vi "GV-ZoomHorizontalDrag.vi"(7 "Gviewer in":refnum<class "Gviewer.lvclass">, 8 "error in (no error)":errorcluster, 10 "Coords":T1, 11 "pict in":picture) -> (0 "error out":errorcluster, 3 "pict out":picture)   [LabVIEW 2020, in "Gviewer.lvclass"]
doc: "Andre Koelewijn, 8 May 2021\n\nDraw the zoom window for Horizontal Area"
uses:
  Gviewer.lvclass
  <vilib>/Utility/miscctls.llb/LVPoint32TypeDef.ctl
  Gviewer.lvclass/Gviewer.ctl
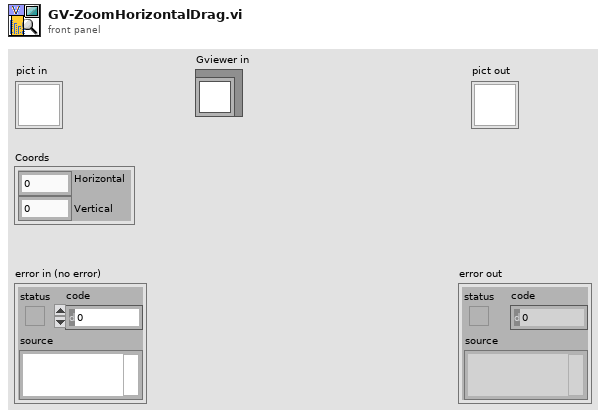
[diagram p1: front panel]
types:
  T1 = typedef "LVPoint32TypeDef.ctl" = cluster{"Horizontal":i32, "Vertical":i32}
  T2 = cluster{"Width":i16, "Style":enum32{"Solid", "Dash", "Dot", "DashDot", "DashDotDot"}}
  T3 = cluster{"left":i16, "top":i16, "right":i16, "bottom":i16}
  T4 = cluster{"horizontal":enum16{"left", "center", "right"}, "vertical":enum16{"top", "center", "bottom"}}
  T5 = typedef "LVRectTypeDef.ctl" = cluster{"Left":i16, "Top":i16, "Right":i16, "Bottom":i16}
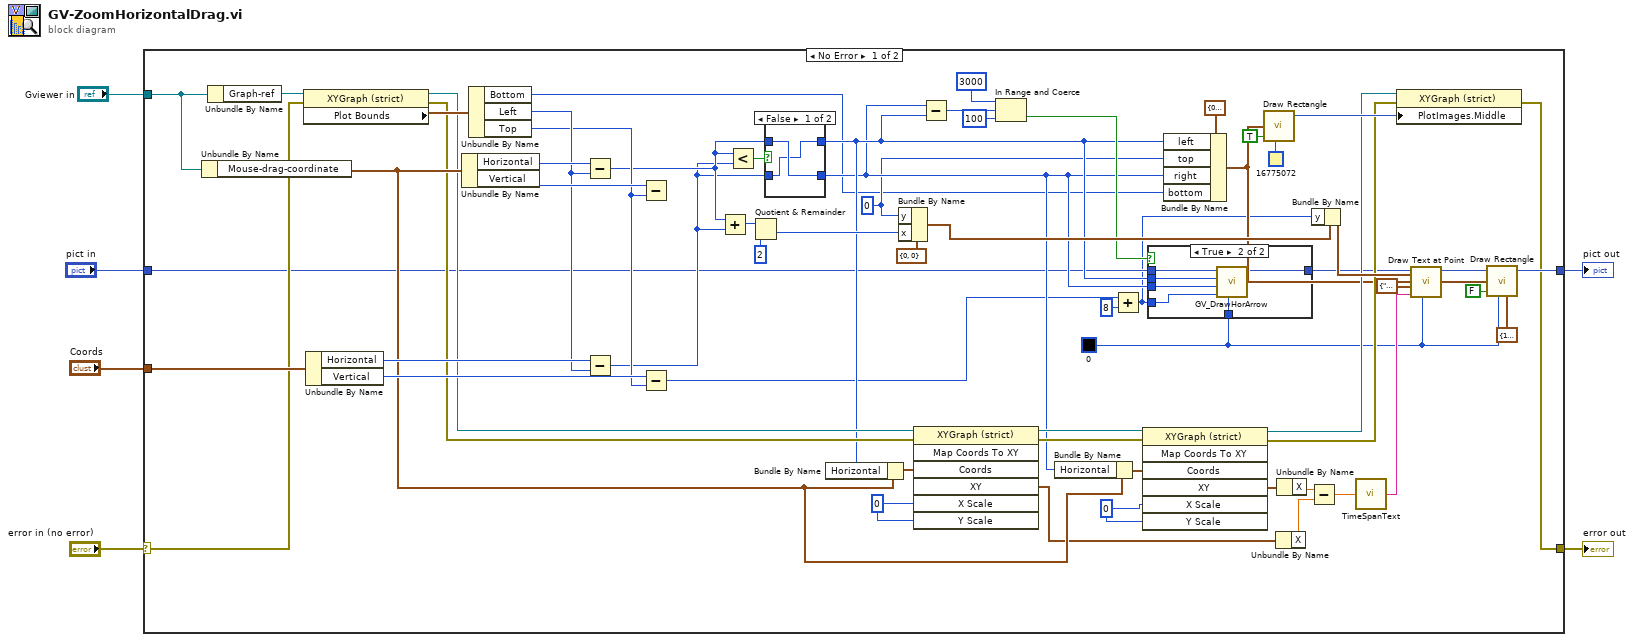
[diagram p0: block diagram]
diagram:
  n1 = case shown="No Error" "error in (no error)" {
    selector: "error in (no error)" -> [w40 w81]
    tunnel: [w28 w81] -> w5
    tunnel: "pict in" -> [w9 w80]
    tunnel: [w51 w80] -> w3
    tunnel: "Coords" -> [w67 _]
    tunnel: "Gviewer in" -> [w49 _]
    frame No Error {
      w10 = u32 0 ("Color")
      w12 = i16 0 ("top")
      w37 = 0 ("X Scale")
      w39 = 0 ("X Scale")
      n2 = Unbundle By Name(w49) -> ("Mouse-drag-coordinate"=w35:T1)
      n3 = Unbundle By Name(w49) -> ("Graph-ref"=w62:refnum<vi>)
      n4 = property class="XYGraph (strict)"(reference=w62, error in=w40) -> (reference out=w32:refnum<vi>, error out=w30:errorcluster, "Plot Bounds"=w61:T5)
      n5 = Unbundle By Name(w67) -> ("Horizontal"=w58:i32, "Vertical"=w56:i32)
      n6 = Unbundle By Name(w35) -> ("Horizontal"=w60:i32, "Vertical"=w59:i32)
      n7 = Unbundle By Name(w61) -> ("Bottom"=w11:i16, "Left"=w57:i16, "Top"=w55:i16)
      n8 = Subtract(x=w60, y=w57) -> (x-y=w48:i32)
      n9 = Subtract(x=w58, y=w57) -> (x-y=w47:i32)
      n10 = Subtract(x=w59, y=w55) -> ()  [unwired: 1 out]
      n11 = Subtract(x=w56, y=w55) -> (x-y=w8:i32)
      n12 = Add(x=w48, y=w47) -> (x+y=w46:i32)
      n13 = Less?(x=w48, y=w47) -> (x < y?=w54:bool)
      n14 = Quotient & Remainder(x=w46, y=2) -> (floor(x/y)=w43:i32)  [unwired: 1 out]
      n15 = case shown="False" w54 {
        tunnel: w48 -> [w77 w79]
        tunnel: [w76 w79] -> w15
        tunnel: [w77 w78] -> w14
        tunnel: w47 -> [w76 w78]
        frame False {
        }
        frame True {
        }
      }
      n16 = Bundle By Name(cluster=w35, "Horizontal"=w15) -> (w38:T1)
      n17 = Bundle By Name(cluster=cluster{"x":i16, "y":i16} {"x"=0, "y"=0} ("origin"), "y"=w12, "x"=w43) -> (w42:cluster{"x":i16, "y":i16})
      n18 = invoke class="XYGraph (strict)" method="Map Coords To XY"(reference=w32, error in=w30, "Coords"=w38, "X Scale"=w39, "Y Scale"=w39) -> (reference out=w36:refnum<vi>, error out=w33:errorcluster, "XY"=w25:cluster{"X":dbl, "Y":dbl})  [unwired: 2 in, 4 out]
      n19 = Subtract(x=w14, y=w15) -> (x-y=w20:i32)
      n20 = In Range and Coerce(upper limit=3000, x=w20, lower limit=100) -> (In Range?=w16:bool)  [unwired: 1 out]
      n21 = Bundle By Name(cluster=w35, "Horizontal"=w14) -> (w34:T1)
      n22 = Add(x=w8, y=8) -> (x+y=w7:i32)
      n23 = invoke class="XYGraph (strict)" method="Map Coords To XY"(reference=w36, error in=w33, "Coords"=w34, "X Scale"=w37, "Y Scale"=w37) -> (reference out=w31:refnum<vi>, error out=w29:errorcluster, "XY"=w27:cluster{"X":dbl, "Y":dbl})  [unwired: 2 in, 4 out]
      n24 = case shown="True" w16 {
        tunnel: w9 -> [w69 w75]
        tunnel: [w69 w74] -> w17
        tunnel: w15 -> [_ w73]
        tunnel: w14 -> [_ w72]
        tunnel: w7 -> [_ w71]
        tunnel: w10 -> [_ w70]
        frame False {
        }
        frame True {
          n25 = call "GV_DrawHorArrow.vi"("Color"=w70, "Vertical"=w71, "Right"=w72, "Left"=w73, "Pict-in"=w75) -> ("Pict-out"=w74:picture)  [unwired: 6 in]
        }
      }
      n26 = Bundle By Name(cluster=T3 {"left"=0, "top"=0, "right"=0, "bottom"=0} ("rect"), "left"=w15, "top"=w12, "right"=w14, "bottom"=w11) -> (w21:T3)
      n27 = call <vilib>:"Draw Rectangle.vi"("rect"=w21, "fill?(F)"=TRUE, "color(black)"=u32 16775072) -> ("new picture"=w66:picture)  [unwired: 6 in]
      n28 = Unbundle By Name(w25) -> ("X"=w24:dbl)
      n29 = Unbundle By Name(w27) -> ("X"=w26:dbl)
      n30 = Subtract(x=w26, y=w24) -> (x-y=w23:dbl)
      n31 = Bundle By Name(cluster=w42, "y"=w7) -> (w41:cluster{"x":i16, "y":i16})
      n32 = call "TimeSpanText.vi"("Timespan"=w23) -> ("TimeSpanText"=w22:string)  [unwired: 4 in]
      n33 = property class="XYGraph (strict)"(reference=w31, error in=w29, "PlotImages.Middle"=w66) -> (error out=w28:errorcluster)  [unwired: 1 out]
      n34 = call <vilib>:"Draw Text at Point.vi"("text color(black)"=w10, "text"=w22, "alignment(left, top)"=T4 {"horizontal"=enum."center", "vertical"=enum."center"}, "origin"=w41, "picture"=w17) -> ("new picture"=w52:picture)  [unwired: 5 in, 1 out]
      n35 = call <vilib>:"Draw Rectangle.vi"("picture"=w52, "rect"=w21, "fill?(F)"=FALSE, "color(black)"=w10, "pen"=T2 {"Width"=1, "Style"=enum."Dot"}) -> ("new picture"=w51:picture)  [unwired: 4 in]
    }
    frame Error {
    }
  }
  "error out" <- w5
  "pict out" <- w3
